vi "Wait.vi"(9 "Target Time (s)":dbl, 11 "First Time?":bool) -> (1 "ElapsedTime":dbl, 3 "Completed":bool)   [LabVIEW 2018]
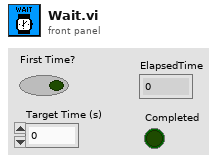
[diagram p1: front panel]
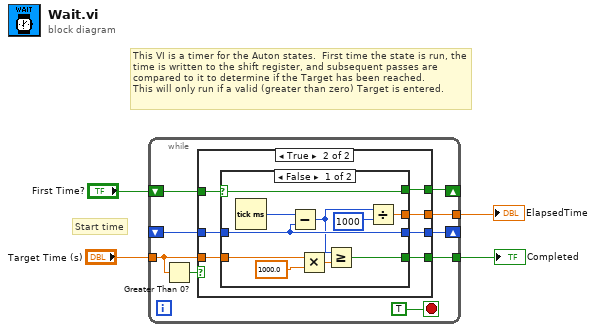
[diagram p0: block diagram]
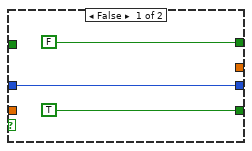
[diagram p2: hidden frame]
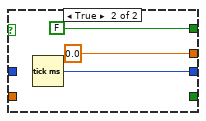
[diagram p3: hidden frame]
diagram:
  # "This VI is a timer for the Auton states.  First time the state is run, the time is written to the shift register, and subsequent passes are compared to it to determine if the Target has been reached.\nThis will only run if a valid (greater than zero) Target is entered."
  # "Start time"
  n1 = while {
    shift-right: [w11] -> _
    shift-left: "First Time?" -> [w12]
    shift-right: [w10] -> _
    shift-left: _ -> [w9]
    tunnel: "Target Time (s)" -> [w5]
    tunnel: [w8] -> w3
    tunnel: [w7] -> w4
    stop <- TRUE stop-if-true
    n2 = Greater Than 0?(x=w5) -> (x > 0?=w6:bool)
    n3 = case shown="True" w6 {
      tunnel: w12 -> [_ w23]
      tunnel: [FALSE w22] -> w11
      tunnel: [w16 w21] -> w10
      tunnel: w9 -> [w16 w20]
      tunnel: w5 -> [_ w19]
      tunnel: [TRUE w18] -> w8
      tunnel: [_ w17] -> w7
      frame False {
      }
      frame True {
        n4 = case shown="False" w23 {
          selector: w23 -> [w33 _]
          tunnel: [w33 FALSE] -> w22
          tunnel: [w31 w35] -> w21
          tunnel: w20 -> [w31 _]
          tunnel: w19 -> [w30 _]
          tunnel: [w27 _] -> w18
          tunnel: [w26 0.0] -> w17
          frame False {
            n5 = Tick Count (ms)() -> (millisecond timer value=w32:u32)
            n6 = Subtract(x=w32, y=w31) -> (x-y=w24:u32)
            n7 = Multiply(x=w30, y=1000.0) -> (x*y=w28:dbl)
            n8 = Greater Or Equal?(x=w24, y=w28) -> (x >= y?=w27:bool)
            n9 = Divide(x=w24, y=u32 1000 ("x")) -> (x/y=w26:dbl)
          }
          frame True {
            n10 = Tick Count (ms)() -> (millisecond timer value=w35:u32)
          }
        }
      }
    }
  }
  "Completed" <- w3
  "ElapsedTime" <- w4
